vi "Test Coffee Shop Add People With Duplicate Names.vi"(8 "error in (no error)":errorcluster, 11 "Coffee Shop Test In":refnum<class "Coffee Shop Test.lvclass">) -> (0 "error out":errorcluster, 3 "Coffee Shop Test Out":refnum<class "Coffee Shop Test.lvclass">)   [LabVIEW 2020, in "Coffee Shop Test.lvclass"]
uses:
  Coffee Shop Test.lvclass
  Coffee Shop/Coffee Shop.lvclass
  <vilib>/Asteme/Triarc Framework/Process/Process.lvclass
  <vilib>/Asteme/LUnit/Test Case.lvclass
  C:/Program Files (x86)/National Instruments/LabVIEW 2020/vi.lib/Asteme/Triarc Framework/Application/Application.lvclass
  C:/Program Files (x86)/National Instruments/LabVIEW 2020/vi.lib/Asteme/Triarc Framework/Process/Process.lvclass
  C:/Program Files (x86)/National Instruments/LabVIEW 2020/vi.lib/Asteme/Triarc Framework/Base/Base.lvclass
  C:/Program Files (x86)/National Instruments/LabVIEW 2020/vi.lib/Asteme/Triarc Framework/Error Handler Interface/Error Handler Interface.lvclass
  C:/Program Files (x86)/National Instruments/LabVIEW 2020/vi.lib/Asteme/Triarc Framework/Logging/Logging.lvclass
  C:/Users/anton/Documents/GitHub/Triarc-Examples/Coffee Shop/Coffee Shop/Coffee Shop.lvclass
  C:/Program Files (x86)/National Instruments/LabVIEW 2020/vi.lib/Asteme/Triarc Framework Test Suite/Application Test/Application Test.lvclass
  C:/Program Files (x86)/National Instruments/LabVIEW 2020/vi.lib/Asteme/Triarc Framework Test Suite/Process Test/Process Test.lvclass
  C:/Program Files (x86)/National Instruments/LabVIEW 2020/vi.lib/Asteme/Triarc Framework Test Suite/Base Class Test/Base Test.lvclass
  C:/Program Files (x86)/National Instruments/LabVIEW 2020/vi.lib/Asteme/LUnit/Test Case.lvclass
  C:/Users/anton/Documents/GitHub/Triarc-Examples/Coffee Shop/Coffee Shop Test/Coffee Shop Test.lvclass
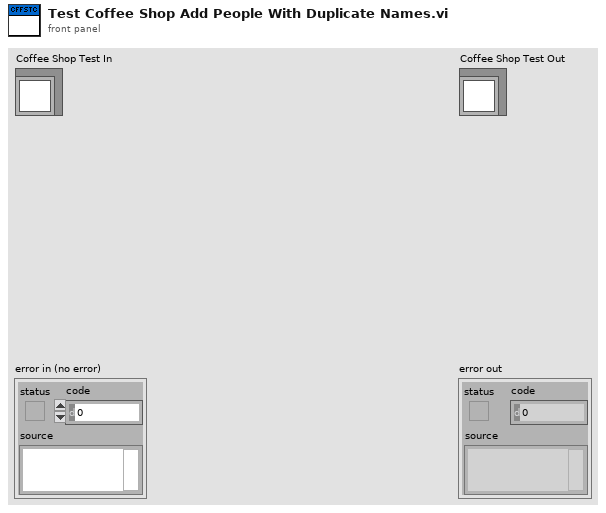
[diagram p1: front panel]
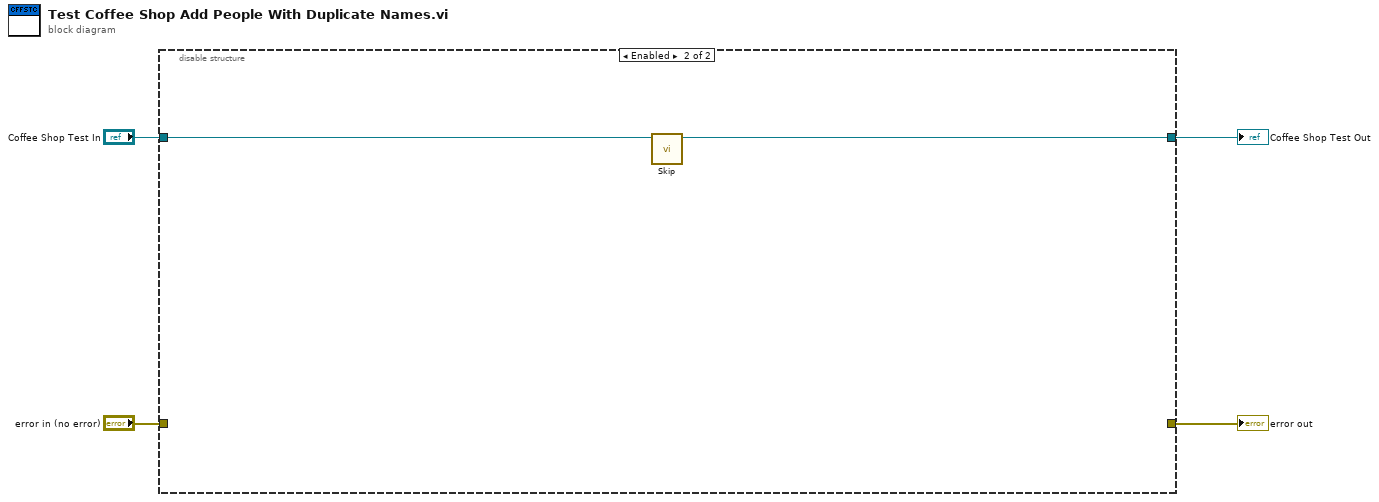
[diagram p0: block diagram]
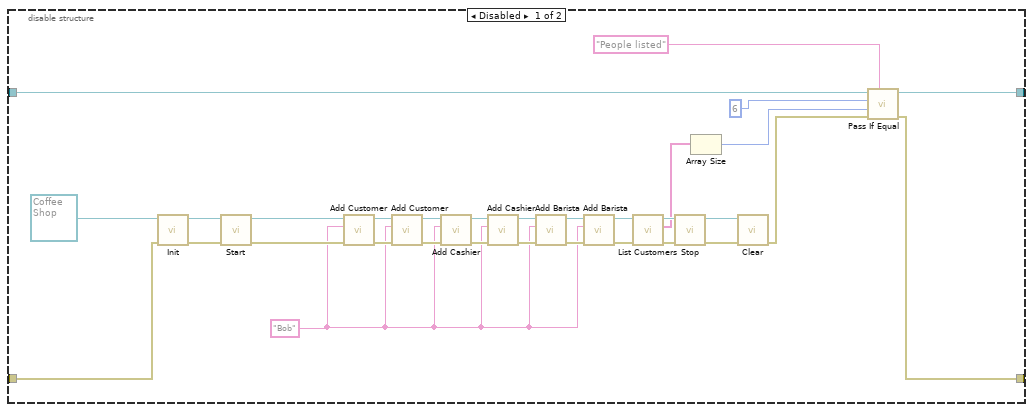
[diagram p2: hidden frame]
diagram:
  n1 = disable-structure shown="Enabled" {
    disable-tunnel: "Coffee Shop Test In" -> [w35 w37]
    disable-tunnel: [w26 w36] -> w3
    disable-tunnel: "error in (no error)" -> [w25 _]
    disable-tunnel: [w23 _] -> w1
    frame Disabled {
      w5 = "Bob" ("Name")
      n2 = call-dynamic "Init.vi"("error in (no error)"=w25, "Process In"=refnum<class "Coffee Shop.lvclass"> refnum ("Coffee Shop.lvclass")) -> ("error out"=w33:errorcluster, "Process Out"=w34:refnum<class "Coffee Shop.lvclass">)  [unwired: 8 in]
      n3 = call <vilib>:"Start.vi"("error in (no error)"=w33, "Process In"=w34) -> ("error out"=w28:errorcluster, "Process Out"=w27:refnum<class "Coffee Shop.lvclass">)  [unwired: 8 in]
      n4 = call "Add Customer.vi"("error in (no error)"=w28, "Name"=w5, "Coffee Shop in"=w27) -> ("error out"=w29:errorcluster, "Coffee Shop out"=w13:refnum<class "Coffee Shop.lvclass">)  [unwired: 7 in]
      n5 = call "Add Customer.vi"("error in (no error)"=w29, "Name"=w5, "Coffee Shop in"=w13) -> ("error out"=w14:errorcluster, "Coffee Shop out"=w12:refnum<class "Coffee Shop.lvclass">)  [unwired: 7 in]
      n6 = call "Add Cashier.vi"("error in (no error)"=w14, "Name"=w5, "Coffee Shop in"=w12) -> ("error out"=w21:errorcluster, "Coffee Shop out"=w10:refnum<class "Coffee Shop.lvclass">)  [unwired: 7 in]
      n7 = call "Add Cashier.vi"("error in (no error)"=w21, "Name"=w5, "Coffee Shop in"=w10) -> ("error out"=w11:errorcluster, "Coffee Shop out"=w9:refnum<class "Coffee Shop.lvclass">)  [unwired: 7 in]
      n8 = call "Add Barista.vi"("error in (no error)"=w11, "Name"=w5, "Coffee Shop in"=w9) -> ("error out"=w15:errorcluster, "Coffee Shop out"=w7:refnum<class "Coffee Shop.lvclass">)  [unwired: 7 in]
      n9 = call "Add Barista.vi"("error in (no error)"=w15, "Name"=w5, "Coffee Shop in"=w7) -> ("error out"=w8:errorcluster, "Coffee Shop out"=w6:refnum<class "Coffee Shop.lvclass">)  [unwired: 7 in]
      n10 = call "List Customers.vi"("error in (no error)"=w8, "Coffee Shop in"=w6) -> ("error out"=w20:errorcluster, "Names"=w18:string[], "Coffee Shop out"=w19:refnum<class "Coffee Shop.lvclass">)  [unwired: 7 in]
      n11 = call <vilib>:"Stop.vi"("error in (no error)"=w20, "Process In"=w19) -> ("error out"=w31:errorcluster, "Process Out"=w32:refnum<class "Coffee Shop.lvclass">)  [unwired: 7 in, 1 out]
      n12 = Array Size(array=w18) -> (size(s)=w17:i32)
      n13 = call-dynamic "Clear.vi"("error in (no error)"=w31, "Application In"=w32) -> ("error out"=w24:errorcluster)  [unwired: 9 in]
      n14 = call <vilib>:"Pass If Equal.vi"("Description"="People listed", "error in (no error)"=w24, "Actual"=w17, "Expected"=6 ("size(s)"), "Test Case In"=w35) -> ("error out"=w23:errorcluster, "Test Case Out"=w26:refnum<class "Coffee Shop Test.lvclass">)  [unwired: 5 in]
    }
    frame Enabled {
      n15 = call <vilib>:"Skip.vi"("Test Case In"=w37) -> ("Test Case Out"=w36:refnum<class "Coffee Shop Test.lvclass">)  [unwired: 9 in, 1 out]
    }
  }
  "error out" <- w1
  "Coffee Shop Test Out" <- w3
